vi "Elevator_Set.vi"() -> ()   [LabVIEW 2018]
uses:
  <vilib>/Rock Robotics/WPI/DriverStation/WPI_DriverStationRobotMode2.ctl
  Elevator_Control_Type.ctl
  Elevator_Enum_States.ctl
  Global_Variables/Elevator_Globals.vi
  Global_Variables/Robot_Global_Data.vi
  Global_Variables/Sensor_Values.vi
  Global_Variables/Autonomous_Globals.vi
  Global_Variables/LED_Globals.vi
panel:
  in  "Climb_Position_Level_Two":dbl=12000.0
  in  "Climb_Position_Level_Three":dbl=33500.0
  out "Cargo_Mode_for_Scoring":bool
  out "Cargo_Mode":bool
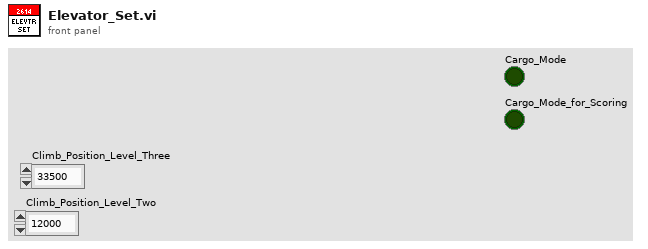
[diagram p1: front panel]
types:
  T1 = typedef "Elevator_Control_Type.ctl" = enum16{"No_Op", "Shift", "Brake", "Manual_Elevator_Up", "Manual_Elevator_Down", "Manual_Climb_Up", "Manual_Climb_Down", "Manual_Position_Control", "Elevator_Retract", "Elevator_Extend", "Brake_In_Climb", "Position_Control", "Position", "Shift_Climb"}
  T2 = typedef "WPI_DriverStationRobotMode2.ctl" = enum16{"Autonomous Disabled", "Autonomous Enabled", "Teleop Disabled", "Teleop Enabled", "Disconnected", "Finish", "Test Disabled", "Test Enabled", "Emergency Stopped"}
  T3 = typedef "Elevator_Enum_States.ctl" = enum16{"Current_Position", "High_Rocket_Hatch_Panel_Floor", "High_Rocket_Hatch_Panel", "Mid_Rocket_Hatch_Panel_Floor", "Mid_Rocket_Hatch_Panel", "Low_Rocket_Hatch_Panel", "Cargo_Ship_Hatch_Panel", "Loading_Station_Hatch_Panel", "Ground_Pickup_Hatch_Panel", "High_Rocket_Cargo", "Mid_Rocket_Cargo", "Low_Rocket_Cargo", "Cargo_Ship_Cargo", "Loading_Station_Cargo", "Ground_Pickup_Cargo", "Depot_Pickup_Cargo", "Descend_Off_Platform", "Stow_Cargo"}
  T4 = typedef "Elevator_Notifier.ctl" = cluster{"Elevator_Control_Type":T1, "Shift":bool, "Brake":bool, "Manual_Lift_Up":bool, "Manual_Lift_Down":bool, "Climb_Advance":bool, "Climb_Reverse":bool, "Low_Rocket":bool, "Mid_Rocket":bool, "High_Rocket":bool, "Cargo_Ship":bool, "Hatch_Floor":bool, "Cargo_Floor":bool, "HP_Hatch":bool, "HP_Cargo":bool, "Depot_Cargo":bool, "Stow":bool, "Set_Position":T3, "Intake_Mode":bool, "Climb_Distance":dbl, "Level_Two":bool, "Parameter_One":dbl, "Parameter_Two":dbl, "Parameter_Three":dbl, "Step":i32, "Elevator_Notifier":refnum<notifier>, "Brake_State":bool, "Shift_State":bool}
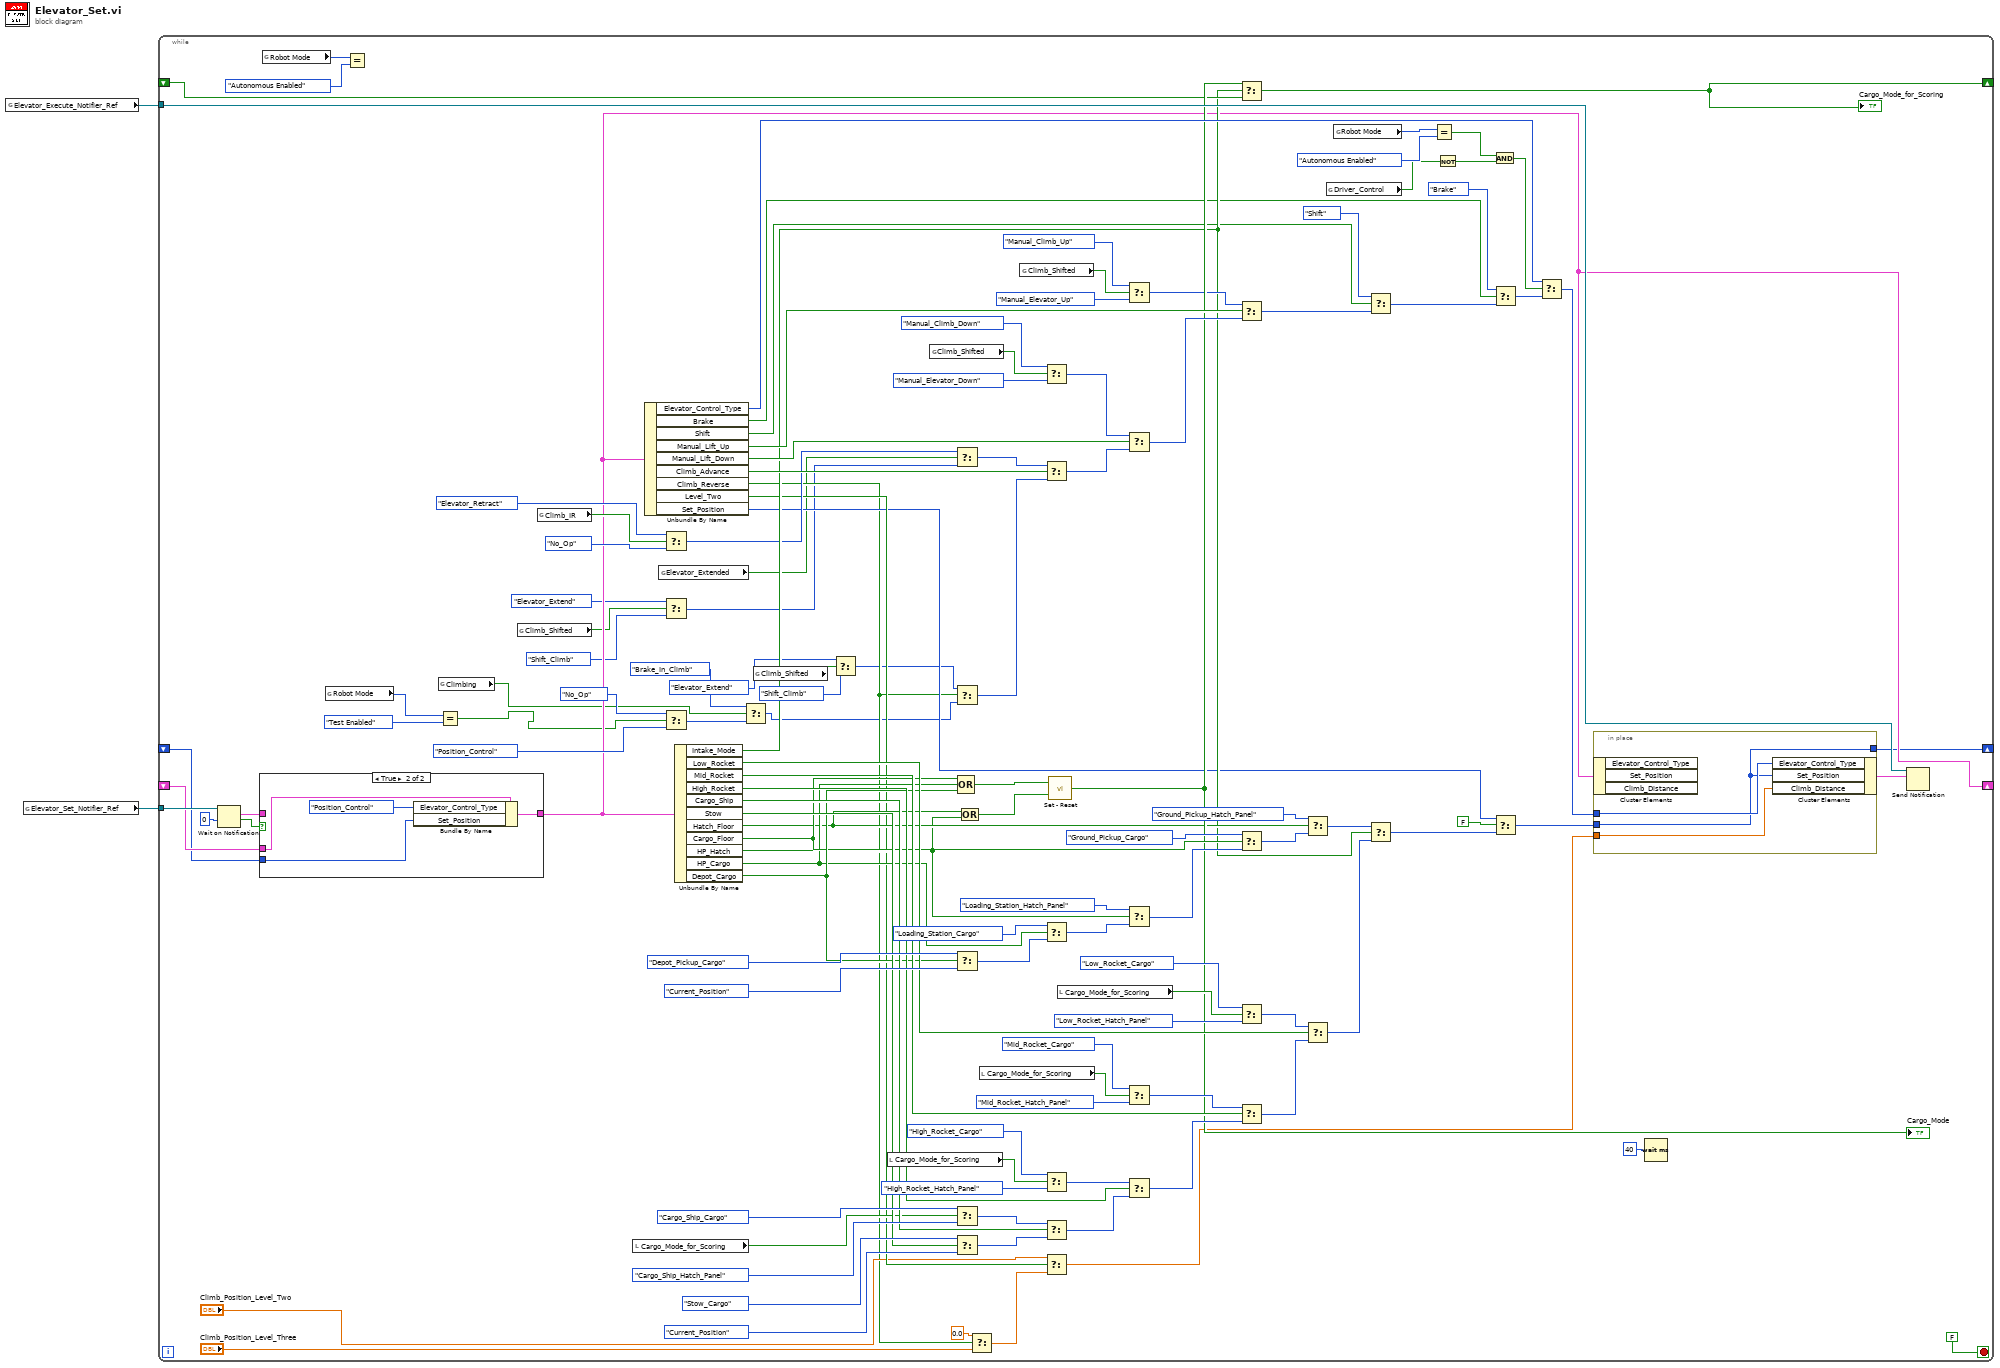
[diagram p0: block diagram]
diagram:
  n1 = global read "Elevator_Globals.vi" "Elevator_Execute_Notifier_Ref"() -> (w1:refnum<notifier>)
  n2 = global read "Elevator_Globals.vi" "Elevator_Set_Notifier_Ref"() -> (w2:refnum<notifier>)
  n3 = while {
    tunnel: w2 -> [w127]
    tunnel: w1 -> [w125]
    shift-right: [w64] -> _
    shift-left: _ -> [w65]
    shift-right: [w33] -> _
    shift-left: _ -> [w32]
    shift-right: [w31] -> _
    shift-left: _ -> [w30]
    stop <- FALSE stop-if-true
    n4 = Wait on Notification(notifier=w127, timeout in ms (-1)=0) -> (notification=w34:T4, timed out?=w36:bool)  [unwired: 2 in, 2 out]
    n5 = case shown="True" w36 {
      tunnel: w34 -> [w130 _]
      tunnel: [w130 w134] -> w33
      tunnel: w32 -> [_ w132]
      tunnel: w30 -> [_ w131]
      frame False {
      }
      frame True {
        n6 = Bundle By Name(cluster=w132, "Elevator_Control_Type"=Elevator_Control_Type."Position_Control", "Set_Position"=w131) -> (w134:T4)
      }
    }
    n7 = global read "Robot_Global_Data.vi" "Robot Mode"() -> (w40:T2)
    n8 = global read "Robot_Global_Data.vi" "Robot Mode"() -> (w116:T2)
    n9 = Equal?(x=w40, y=WPI_DriverStationRobotMode2."Autonomous Enabled") -> ()  [unwired: 1 out]
    n10 = global read "LED_Globals.vi" "Climbing"() -> (w4:bool)
    n11 = Equal?(x=w116, y=WPI_DriverStationRobotMode2."Test Enabled") -> (x = y?=w7:bool)
    n12 = global read "Elevator_Globals.vi" "Climb_Shifted"() -> (w18:bool)
    n13 = global read "Sensor_Values.vi" "Climb_IR"() -> (w47:bool)
    n14 = local read "Cargo_Mode_for_Scoring"() -> (w70:bool)
    n15 = Unbundle By Name(w33) -> ("Elevator_Control_Type"=w122:T1, "Brake"=w23:bool, "Shift"=w24:bool, "Manual_Lift_Up"=w112:bool, "Manual_Lift_Down"=w111:bool, "Climb_Advance"=w110:bool, "Climb_Reverse"=w27:bool, "Level_Two"=w43:bool, "Set_Position"=w37:T3)
    n16 = global read "Elevator_Globals.vi" "Elevator_Extended"() -> (w22:bool)
    n17 = Select(t=Elevator_Control_Type."Elevator_Retract", s=w47, f=Elevator_Control_Type."No_Op") -> (s? t:f=w48:T1)
    n18 = Select(t=Elevator_Control_Type."Elevator_Extend", s=w18, f=Elevator_Control_Type."Shift_Climb") -> (s? t:f=w20:T1)
    n19 = Select(t=Elevator_Control_Type."No_Op", s=w7, f=Elevator_Control_Type."Position_Control") -> (s? t:f=w6:T1)
    n20 = Unbundle By Name(w33) -> ("Intake_Mode"=w50:bool, "Low_Rocket"=w80:bool, "Mid_Rocket"=w79:bool, "High_Rocket"=w78:bool, "Cargo_Ship"=w77:bool, "Stow"=w76:bool, "Hatch_Floor"=w53:bool, "Cargo_Floor"=w74:bool, "HP_Hatch"=w52:bool, "HP_Cargo"=w73:bool, "Depot_Cargo"=w75:bool)
    n21 = Select(t=Elevator_Control_Type."Brake_In_Climb", s=w4, f=w6) -> (s? t:f=w5:T1)
    n22 = global read "Elevator_Globals.vi" "Climb_Shifted"() -> (w10:bool)
    n23 = Select(t=Elevator_Control_Type."Elevator_Extend", s=w10, f=Elevator_Control_Type."Shift_Climb") -> (s? t:f=w9:T1)
    n24 = local read "Cargo_Mode_for_Scoring"() -> (w69:bool)
    n25 = global read "Elevator_Globals.vi" "Climb_Shifted"() -> (w63:bool)
    n26 = Select(t=w48, s=w22, f=w20) -> (s? t:f=w49:T1)
    n27 = Select(t=w9, s=w27, f=w5) -> (s? t:f=w29:T1)
    n28 = Select(t=Elevator_Enum_States."Depot_Pickup_Cargo", s=w75, f=Elevator_Enum_States."Current_Position") -> (s? t:f=w84:T3)
    n29 = Select(t=Elevator_Enum_States."Cargo_Ship_Cargo" ("f"), s=w70, f=Elevator_Enum_States."Cargo_Ship_Hatch_Panel") -> (s? t:f=w102:T3)
    n30 = Select(t=Elevator_Enum_States."Stow_Cargo", s=w76, f=Elevator_Enum_States."Current_Position" ("Set_Position")) -> (s? t:f=w91:T3)
    n31 = Compound Arithmetic op=OR(w74, w73, w75) -> (w72:bool)
    n32 = Compound Arithmetic op=OR(w53, w52) -> (w71:bool)
    n33 = Select(t=0.0, s=w27, f="Climb_Position_Level_Three") -> (s? t:f=w25:dbl)
    n34 = local read "Cargo_Mode_for_Scoring"() -> (w68:bool)
    n35 = global read "Elevator_Globals.vi" "Climb_Shifted"() -> (w57:bool)
    n36 = Select(t=Elevator_Control_Type."Manual_Climb_Down", s=w63, f=Elevator_Control_Type."Manual_Elevator_Down") -> (s? t:f=w62:T1)
    n37 = Select(t=w49, s=w110, f=w29) -> (s? t:f=w109:T1)
    n38 = Select(t=Elevator_Enum_States."Loading_Station_Cargo", s=w73, f=w84) -> (s? t:f=w85:T3)
    n39 = Select(t=Elevator_Enum_States."High_Rocket_Cargo" ("f"), s=w69, f=Elevator_Enum_States."High_Rocket_Hatch_Panel") -> (s? t:f=w101:T3)
    n40 = Select(t=w102, s=w77, f=w91) -> (s? t:f=w90:T3)
    n41 = Select(t="Climb_Position_Level_Two", s=w43, f=w25) -> (s? t:f=w44:dbl)
    n42 = call "Set - Reset.vi"("Reset"=w71, "Set"=w72) -> ("Output"=w66:bool)
    "Cargo_Mode" <- w66
    n43 = local read "Cargo_Mode_for_Scoring"() -> (w67:bool)
    n44 = Select(t=Elevator_Control_Type."Manual_Climb_Up", s=w57, f=Elevator_Control_Type."Manual_Elevator_Up" ("t")) -> (s? t:f=w59:T1)
    n45 = Select(t=w62, s=w111, f=w109) -> (s? t:f=w113:T1)
    n46 = Select(t=Elevator_Enum_States."Loading_Station_Hatch_Panel", s=w52, f=w85) -> (s? t:f=w86:T3)
    n47 = Select(t=Elevator_Enum_States."Mid_Rocket_Cargo", s=w68, f=Elevator_Enum_States."Mid_Rocket_Hatch_Panel") -> (s? t:f=w100:T3)
    n48 = Select(t=w101, s=w78, f=w90) -> (s? t:f=w89:T3)
    n49 = Select(t=w66, s=w50, f=w65) -> (s? t:f=w64:bool)
    "Cargo_Mode_for_Scoring" <- w64
    n50 = Select(t=w59, s=w112, f=w113) -> (s? t:f=w114:T1)
    n51 = Select(t=Elevator_Enum_States."Ground_Pickup_Cargo", s=w74, f=w86) -> (s? t:f=w87:T3)
    n52 = Select(t=Elevator_Enum_States."Low_Rocket_Cargo", s=w67, f=Elevator_Enum_States."Low_Rocket_Hatch_Panel" ("t")) -> (s? t:f=w103:T3)
    n53 = Select(t=w100, s=w79, f=w89) -> (s? t:f=w88:T3)
    n54 = Select(t=Elevator_Enum_States."Ground_Pickup_Hatch_Panel", s=w53, f=w87) -> (s? t:f=w82:T3)
    n55 = Select(t=w103, s=w80, f=w88) -> (s? t:f=w81:T3)
    n56 = global read "Autonomous_Globals.vi" "Driver_Control"() -> (w14:bool)
    n57 = global read "Robot_Global_Data.vi" "Robot Mode"() -> (w124:T2)
    n58 = Select(t=Elevator_Control_Type."Shift", s=w24, f=w114) -> (s? t:f=w121:T1)
    n59 = Select(t=w82, s=w50, f=w81) -> (s? t:f=w39:T3)
    n60 = Equal?(x=w124, y=WPI_DriverStationRobotMode2."Autonomous Enabled") -> (x = y?=w13:bool)
    n61 = Not(x=w14) -> (.not. x?=w15:bool)
    n62 = And(x=w13, y=w15) -> (x .and. y?=w12:bool)
    n63 = Select(t=Elevator_Control_Type."Brake", s=w23, f=w121) -> (s? t:f=w118:T1)
    n64 = Select(t=w37, s=FALSE, f=w39) -> (s? t:f=w38:T3)
    n65 = Select(t=w122, s=w12, f=w118) -> (s? t:f=w117:T1)
    n66 = in-place {
      in-place-border: w117 -> [w137]
      in-place-border: w44 -> [w136]
      in-place-border: w38 -> [w135]
      in-place-border: [w135] -> w31
      n67 = in-place-cluster #1(w33) -> ()  [unwired: 3 out]
      n68 = in-place-cluster #1("Elevator_Control_Type"=w137, "Set_Position"=w135, "Climb_Distance"=w136) -> (w126:T4)
    }
    n69 = Wait (ms)(milliseconds to wait=u32 40) -> ()  [unwired: 1 out]
    n70 = Send Notification(notification=w126, notifier=w125) -> ()  [unwired: 1 in, 2 out]
  }
